vi "CANOpen_Main_Read TPDOs.vi"(8 "error in (no error)":errorcluster, 9 "Initial Data Array":dbl[](array[numeric])=[0.0, 0.0, 0.0, 0.0], 10 "Nodes":T4[](array[typedef]) {"NMT"."Node init static SDO state" items=["start remote node"=1, "enter pre-operational"=128]; "NMT"."Node run state" items=["start remote node"=1, "stop remote node"=2, "enter pre-operational"=128, "reset node"=129, "reset communication"=130]; "Dynamic SDOs"."Sub-Index (0)" format="%.0x"; "Dynamic SDOs"."Object Index" format="%.0x"; "Dynamic SDOs"."Block Data" format="%.0x"; "RPDOs"."PDO Channel" items=["PDO 1", "PDO 2", "PDO 3", "PDO 4"]; "RPDOs"."Parameters"."Bit Offset" max=8 step=1; "RPDOs"."Parameters"."Byte Offset" max=8 step=1; "TPDOs"."PDO Channel" items=["PDO 1", "PDO 2", "PDO 3", "PDO 4"]; "TPDOs"."Parameters"."Bit Offset" max=8 step=1; "TPDOs"."Parameters"."Byte Offset" max=8 step=1; "SDOs"."Sub-Index (0)" format="%.0x"; "SDOs"."Object Index" format="%.0x"; "SDOs"."Block Data" format="%.0x"}, 11 "xPDO Refs":T1) -> (0 "error out":errorcluster, 1 "Data Array":dbl[](array[numeric]), 3 "New Data?":bool)   [LabVIEW 2013]
uses:
  SubVIS/CANOpen_Node Message Settings.ctl
  Shared Code/CANOpen_PDO Settings.ctl
  Shared Code/CANOpen_PDO Parameter Settings.ctl
  Shared Code/CANOpen_PDO Data Type.ctl
  System Explorer/SubVIs/CANopen Byte Order.ctl
  Shared Code/CANOpen_SDO Settings.ctl
  SubVIS/CANOpen_NMT Settings.ctl
  CanOpen_NMT_Config.ctl
  CanOpen_NMT_Static detect.ctl
  CANOpen_xPDO Refs.ctl
  CanOpen_RPDO Refs.ctl
  CanOpen_TPDO Refs.ctl
  CANOpen Addon Custom Device.lvlib
panel:
  # "LSB"
  # "MSB"
  # "LSB"
  # "MSB"
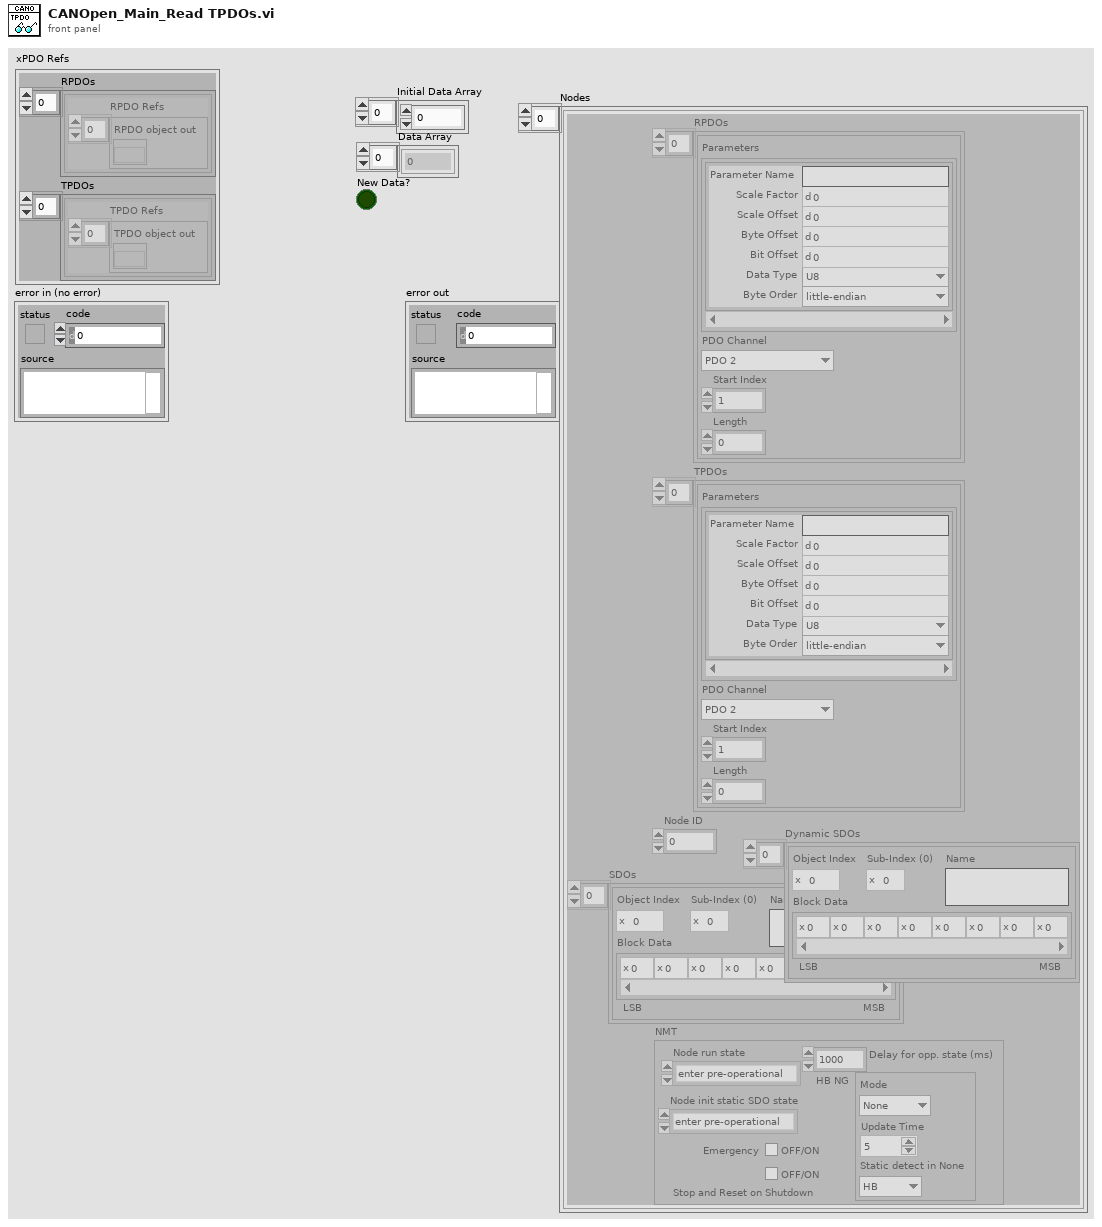
[diagram p1: front panel]
types:
  T1 = typedef "CANOpen_xPDO Refs.ctl" = cluster{"RPDOs":T2[], "TPDOs":T3[]}
  T2 = typedef "CanOpen_RPDO Refs.ctl" = cluster{"RPDO Refs":refnum<k20>[]}
  T3 = typedef "CanOpen_TPDO Refs.ctl" = cluster{"TPDO Refs":refnum<k20>[]}
  T4 = typedef "CANOpen_Node Message Settings.ctl" = cluster{"RPDOs":T5[], "TPDOs":T5[], "Node ID":u8, "SDOs":T9[], "Dynamic SDOs":T9[], "NMT":T10}
  T5 = typedef "CANOpen Addon Custom Device.lvlib/CANOpen_PDO Settings.ctl" = cluster{"Parameters":T6[], "PDO Channel":u8, "Start Index":u32, "Length":u32}
  T6 = typedef "CANOpen Addon Custom Device.lvlib/CANOpen_PDO Parameter Settings.ctl" = cluster{"Parameter Name":string, "Scale Factor":dbl, "Scale Offset":dbl, "Byte Offset":u8, "Bit Offset":u8, "Data Type":T7, "Byte Order":T8}
  T7 = typedef "CANOpen Addon Custom Device.lvlib/CANOpen_PDO Data Type.ctl" = enum16{"U8", "U16", "U32", "I8", "I16", "I32", "Single", "Double", "Boolean"}
  T8 = typedef "CANOpen Addon Custom Device.lvlib/CANopen Byte Order.ctl" = enum16{"big-endian network order", "little-endian"}
  T9 = typedef "CANOpen Addon Custom Device.lvlib/CANOpen_SDO Settings.ctl" = cluster{"Object Index":u16, "Sub-Index (0)":u8, "Block Data":u8[], "Name":string}
  T10 = typedef "CANOpen Addon Custom Device.lvlib/CANOpen_NMT Settings.ctl" = cluster{"Node run state":u16, "Emergency":bool, "HB NG":T11, "Delay for opp. state (ms)":dbl, "Node init static SDO state":u16, "Stop and Reset on Shutdown":bool}
  T11 = typedef "CANOpen Addon Custom Device.lvlib/CanOpen_NMT_Config.ctl" = cluster{"Mode":T12, "Update Time":u16, "Static detect in None":T12}
  T12 = typedef "CANOpen Addon Custom Device.lvlib/CanOpen_NMT_Static detect.ctl" = enum16{"None", "HB", "NG"}
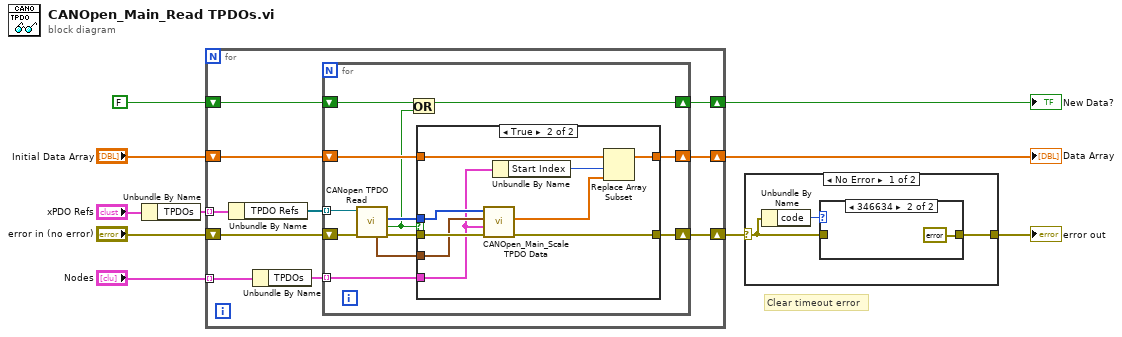
[diagram p0: block diagram]
diagram:
  # "Clear timeout error"
  n1 = Unbundle By Name("xPDO Refs") -> ("TPDOs"=w7:T3[])
  n2 = for {
    tunnel: "Nodes" -> [w11] mode=indexing
    shift-right: [w19] -> w2
    shift-left: "error in (no error)" -> [w20]
    tunnel: w7 -> [w17] mode=indexing
    shift-right: [w14] -> w5
    shift-left: "Initial Data Array" -> [w15]
    shift-right: [w13] -> w3
    shift-left: FALSE -> [w12]
    n3 = Unbundle By Name(w17) -> ("TPDO Refs"=w16:refnum<k20>[])
    n4 = Unbundle By Name(w11) -> ("TPDOs"=w18:T5[])
    n5 = for {
      tunnel: w16 -> [w30] mode=indexing
      shift-right: [w28] -> w19
      shift-left: w20 -> [w29]
      tunnel: w18 -> [w26] mode=indexing
      shift-right: [w24] -> w14
      shift-left: w15 -> [w25]
      shift-right: [w22] -> w13
      shift-left: w12 -> [w21]
      n6 = call <vilib>:"CANopen TPDO Read.vi"("error in (no error)"=w29, "TPDO object in"=w30) -> ("error out"=w32:errorcluster, "new data?"=w23:bool, "data"=w31:u8[], "timestamp"=w27:timestamp)  [unwired: 5 in, 1 out]
      n7 = Or(x=w21, y=w23) -> (x .or. y?=w22:bool)
      n8 = case shown="True" w23 {
        tunnel: w32 -> [w34 w43]
        tunnel: w31 -> [_ w42]
        tunnel: [w34 w41] -> w28
        tunnel: w27 -> [_ w40]
        tunnel: w26 -> [_ w36]
        tunnel: w25 -> [w33 w39]
        tunnel: [w33 w37] -> w24
        frame False {
        }
        frame True {
          n9 = call "CANOpen_Main_Scale TPDO Data.vi"("error in (no error)"=w43, "PDO Settings"=w36, "timestamp"=w40, "data"=w42) -> ("error out"=w41:errorcluster, "Array"=w38:dbl[])  [unwired: 5 in, 1 out]
          n10 = Unbundle By Name(w36) -> ("Start Index"=w35:u32)
          n11 = Replace Array Subset(array=w39, new element=w38, index=w35) -> (w37:dbl[])
        }
      }
    }
  }
  "Data Array" <- w5
  "New Data?" <- w3
  n12 = case shown="No Error" w2 {
    selector: w2 -> [w44 w49]
    tunnel: [w45 w49] -> w1
    frame No Error {
      n13 = Unbundle By Name(w44) -> ("code"=w46:i32)
      n14 = case shown="346634" w46 {
        tunnel: [w47 errorcluster {"status"=FALSE, "code"=0, "source"=""} ("error IO")] -> w45
        tunnel: w44 -> [w47 _]
        frame 0, Default {
        }
        frame 346634 {
        }
      }
    }
    frame Error {
    }
  }
  "error out" <- w1
